vi "Solve1.vi"(8 "Error In":errorcluster, 11 "object in":refnum<class "2021_9.lvclass">) -> (0 "Error Out":errorcluster, 2 "Result":u64, 3 "object out":refnum<class "2021_9.lvclass">)   [LabVIEW 2020, in "2021_9.lvclass"]
uses:
  2021_9.lvclass
  2021_9.lvclass/2021_9.ctl
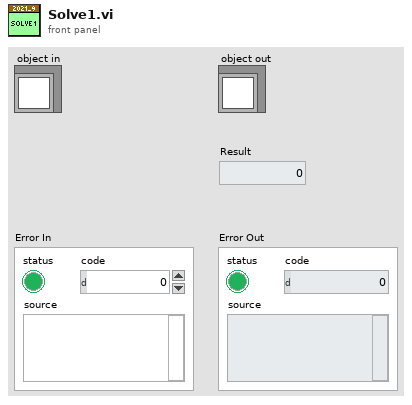
[diagram p1: front panel]
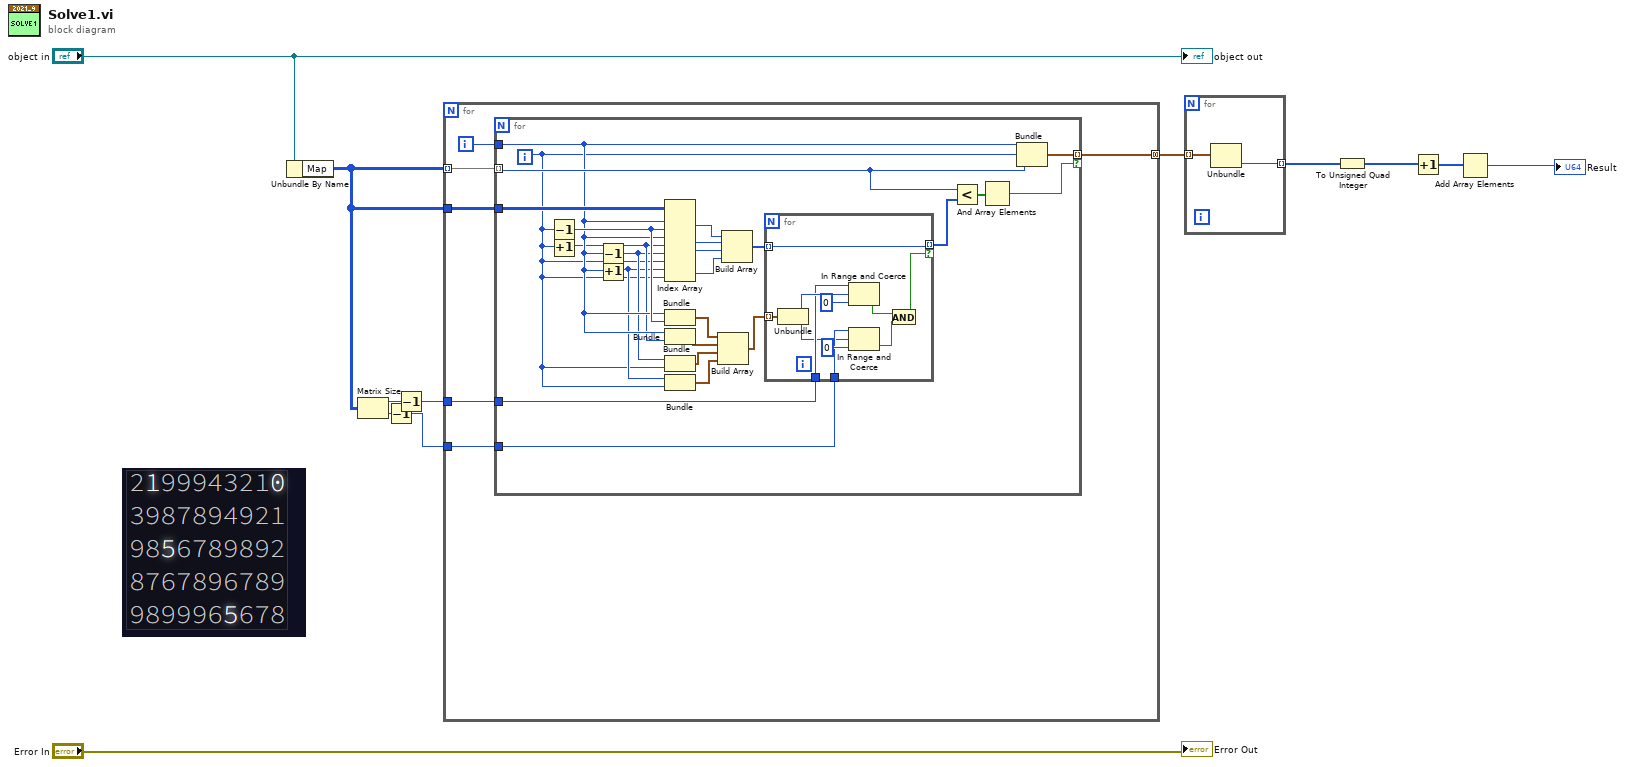
[diagram p0: block diagram]
diagram:
  n1 = Unbundle By Name("object in") -> ("Map"=w10:u8[][])
  n2 = Matrix Size(0:w10) -> (1:w8:i32, 2:w7:i32)
  n3 = Decrement(x=w7) -> (x-1=w6:i32)
  n4 = Decrement(x=w8) -> (x-1=w9:i32)
  n5 = for {
    tunnel: w10 -> [w18] mode=indexing
    tunnel: [w16] -> w5 mode=concatenating
    tunnel: w10 -> [w15]
    tunnel: w9 -> [w14]
    tunnel: w6 -> [w13]
    i -> [w17]
    n6 = for {
      tunnel: w18 -> [w41] mode=indexing
      tunnel: w17 -> [w37]
      tunnel: [w42] -> w16 mode=indexing if=w40
      tunnel: w15 -> [w39]
      tunnel: w14 -> [w20]
      tunnel: w13 -> [w19]
      i -> [w33]
      n7 = Decrement(x=w33) -> (x-1=w38:i32)
      n8 = Increment(x=w33) -> (x+1=w36:i32)
      n9 = Decrement(x=w37) -> (x-1=w35:i32)
      n10 = Increment(x=w37) -> (x+1=w34:i32)
      n11 = Index Array(array=w39, index (row) #1=w37, index (col) #1=w38, index (row) #2=w37, index (col) #2=w36, index (row) #3=w35, index (col) #3=w33, index (row) #4=w34, index (col) #4=w33) -> (element #1=w28:u8, element #2=w27:u8, element #3=w26:u8, element #4=w25:u8)
      n12 = Bundle(w37, w38) -> (w32:cluster{i32, i32})  [unwired: 1 in]
      n13 = Bundle(w37, w36) -> (w31:cluster{i32, i32})  [unwired: 1 in]
      n14 = Bundle(w35, w33) -> (w30:cluster{i32, i32})  [unwired: 1 in]
      n15 = Bundle(w34, w33) -> (w29:cluster{i32, i32})  [unwired: 1 in]
      n16 = Build Array(w32, w31, w30, w29) -> (w21:cluster{i32, i32}[])
      n17 = Build Array(w28, w27, w26, w25) -> (w24:u8[])
      n18 = for {
        tunnel: w24 -> [w53] mode=indexing
        tunnel: [w53] -> w23 mode=indexing if=w43
        tunnel: w21 -> [w50] mode=indexing
        tunnel: w20 -> [w48]
        tunnel: w19 -> [w47]
        n19 = Unbundle(w50) -> (w49:i32, w46:i32)
        n20 = In Range and Coerce(upper limit=w48, x=w49, lower limit=0) -> (In Range?=w45:bool)  [unwired: 1 out]
        n21 = In Range and Coerce(upper limit=w47, x=w46, lower limit=0) -> (In Range?=w44:bool)  [unwired: 1 out]
        n22 = And(x=w45, y=w44) -> (x .and. y?=w43:bool)
      }
      n23 = Less?(x=w41, y=w23) -> (x < y?=w22:bool[])
      n24 = And Array Elements(Boolean array=w22) -> (logical AND=w40:bool)
      n25 = Bundle(w37, w33, w41) -> (w42:cluster{i32, i32, u8})  [unwired: 1 in]
    }
  }
  n26 = for {
    tunnel: w5 -> [w55] mode=indexing
    tunnel: [w54] -> w4 mode=indexing
    n27 = Unbundle(w55) -> (w54:u8)  [unwired: 2 out]
  }
  n28 = To Unsigned Quad Integer(1:w4) -> (0:w1:u64[])
  n29 = Increment(x=w1) -> (x+1=w3:u64[])
  n30 = Add Array Elements(numeric array=w3) -> (sum=→"Result":u64)
  "Error Out" <- "Error In"
  "object out" <- "object in"
